vi "open_dev3.vi"(4 "ViStatus":T2, 7 "InterfaceInfo 2":T3) -> (0 "ViStatus 2":T2, 1 "drv_name":string, 2 "ModuleInfo":T1 {"DacScaleCoef" format="%#_2g"; "DacOffsetCoef" format="%#_2g"}, 3 "InterfaceInfo":T3)   [LabVIEW 2010]
uses:
  Rtusbapi.llb/3000pars.vi
  wrRtusbapi.dll
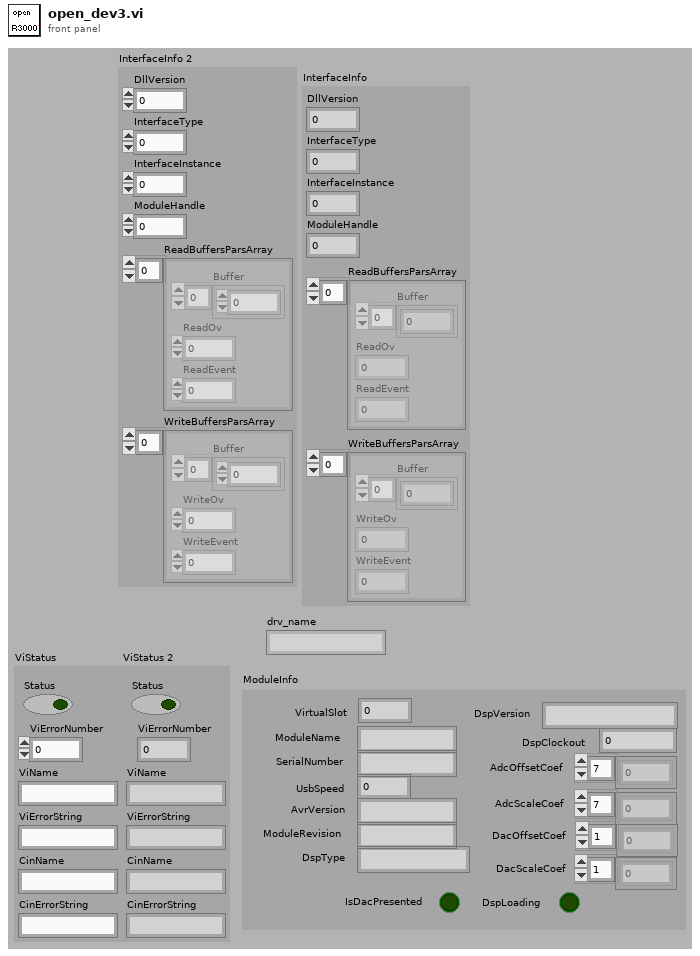
[diagram p1: front panel]
types:
  T1 = cluster{"VirtualSlot":u16, "ModuleName":string, "SerialNumber":string, "UsbSpeed":u8, "AvrVersion":string, "ModuleRevision":string, "DspType":string, "IsDacPresented":bool, "DspLoading":bool, "DspVersion":string, "DspClockout":u32, "AdcOffsetCoef":sgl[], "AdcScaleCoef":sgl[], "DacOffsetCoef":sgl[], "DacScaleCoef":sgl[]}
  T2 = cluster{"Status":bool, "ViErrorNumber":u32, "ViName":string, "ViErrorString":string, "CinName":string, "CinErrorString":string}
  T3 = cluster{"DllVersion":u32, "InterfaceType":u32, "InterfaceInstance":u32, "ModuleHandle":u32, "ReadBuffersParsArray":cluster{"Buffer":i16[], "ReadOv":u32, "ReadEvent":u32}[], "WriteBuffersParsArray":cluster{"Buffer":i16[], "WriteOv":u32, "WriteEvent":u32}[]}
  T4 = cluster{"CRC16":u16, "size":u16, "SerialNumber":string, "Name":string, "Revision":string, "DSPType":string, "IsDACPresent":u16, "DSPClockout":u32, "ADCOffset":sgl[], "ADCScale":sgl[], "DACOffset":sgl[], "DACScale":sgl[]}
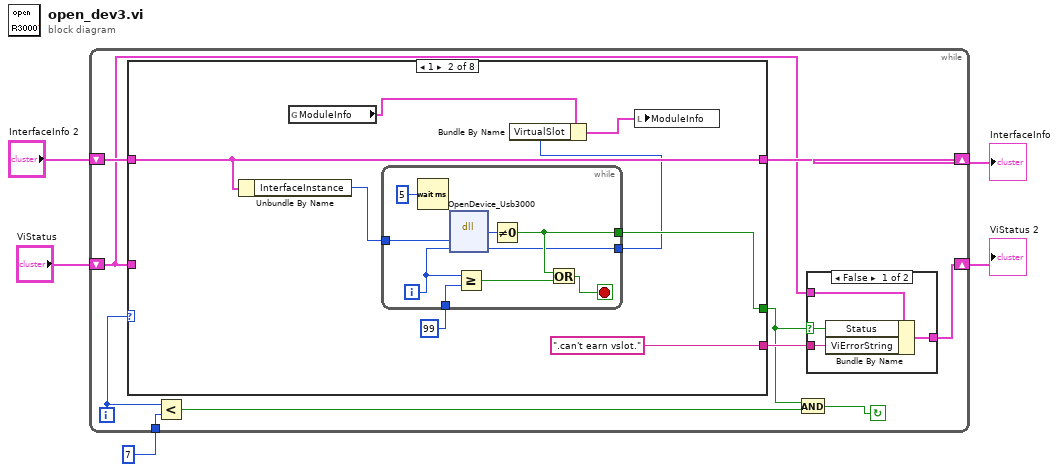
[diagram p0: block diagram]
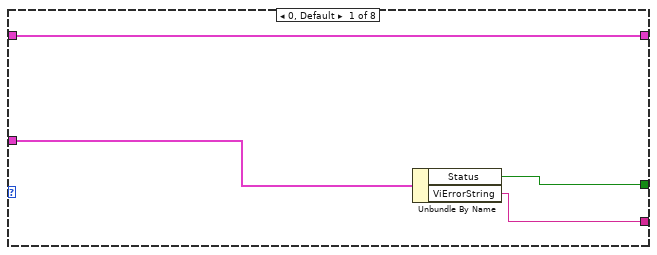
[diagram p3: hidden frame]
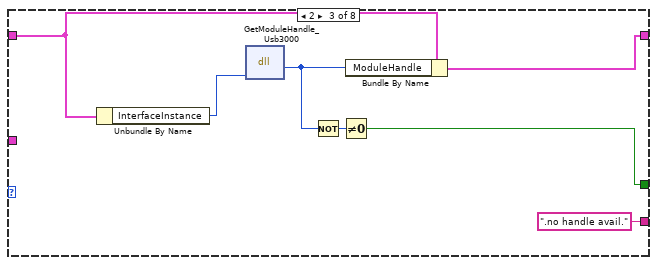
[diagram p4: hidden frame]
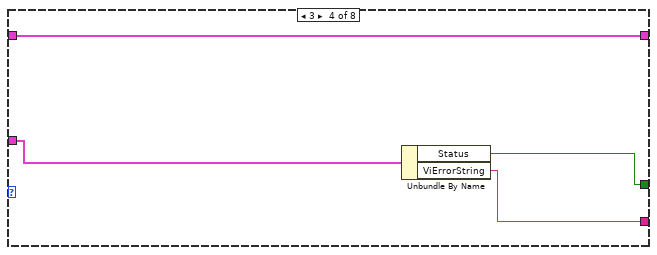
[diagram p5: hidden frame]
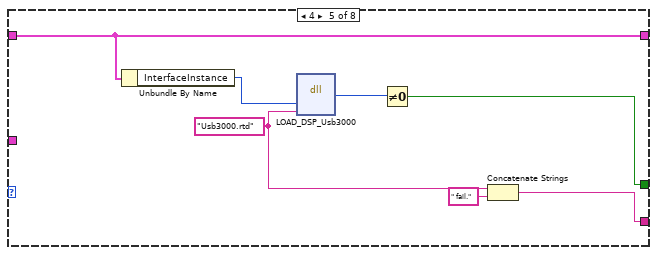
[diagram p6: hidden frame]
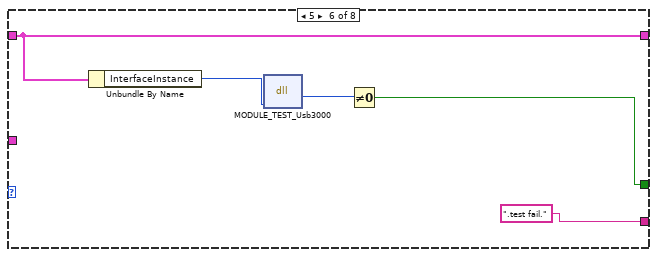
[diagram p7: hidden frame]
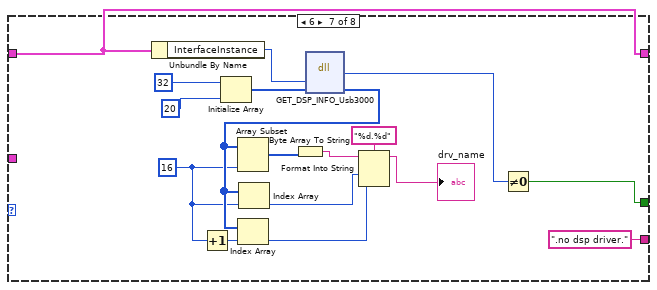
[diagram p8: hidden frame]
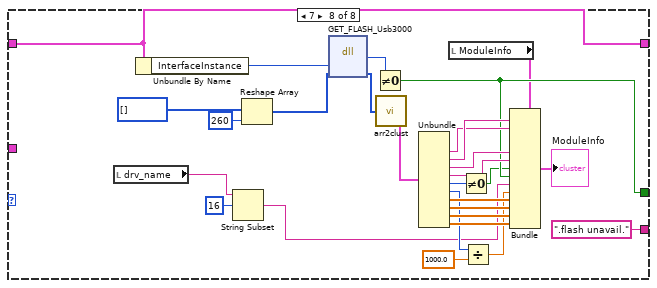
[diagram p9: hidden frame]
diagram:
  n1 = while {
    shift-right: [w14] -> w3
    shift-left: "InterfaceInfo 2" -> [w15]
    shift-right: [w12] -> w2
    shift-left: "ViStatus" -> [w13]
    tunnel: 7 ("y") -> [w6]
    i -> [w10]
    stop <- w7 continue-if-true
    n2 = case shown="1" w10 {
      tunnel: w15 -> [w24 w31 w47 w52 w59 w61 w78 w109]
      tunnel: [w24 w31 w46 w52 w59 w61 w78 w109] -> w14
      tunnel: w13 -> [w23 _ _ w50 _ _ _ _]
      tunnel: [w22 w30 w44 w51 w56 w62 w75 w95] -> w9
      tunnel: [w21 ".can't earn vslot." ("ViErrorString") ".no handle avail." ("ViErrorString") w49 w54 ".test fail." ("ViErrorString") ".no dsp driver." ("ViErrorString") ".flash unavail." ("ViErrorString")] -> w11
      frame 0, Default {
        n3 = Unbundle By Name(w23) -> ("Status"=w22:bool, "ViErrorString"=w21:string)
      }
      frame 1 {
        n4 = Unbundle By Name(w31) -> ("InterfaceInstance"=w32:u32)
        n5 = global read "3000pars.vi" "ModuleInfo"() -> (w26:T1)
        n6 = while {
          tunnel: w32 -> [w41]
          tunnel: [w37] -> w30
          tunnel: 99 -> [w38]
          tunnel: [w34] -> w27
          i -> [w39]
          stop <- w36 stop-if-true
          n7 = Wait (ms)(milliseconds to wait=u32 5) -> ()  [unwired: 1 out]
          n8 = dll-call lib="D:/Work/SibNIIE/SMGR/prj1_pdv_usb/pdv_usb/wrRtusbapi.dll" fn="OpenDevice_Usb3000"(w41, w39) -> (w40:i32, w34:u16)  [unwired: 4 in, 2 out]
          n9 = Greater Or Equal?(x=w39, y=w38) -> (x >= y?=w35:bool)
          n10 = Not Equal To 0?(x=w40) -> (x != 0?=w37:bool)
          n11 = Or(x=w37, y=w35) -> (x .or. y?=w36:bool)
        }
        n12 = Bundle By Name(cluster=w26, "VirtualSlot"=w27) -> (w25:T1)
        n13 = local write "ModuleInfo"(w25) -> ()
      }
      frame 2 {
        n14 = Unbundle By Name(w47) -> ("InterfaceInstance"=w48:u32)
        n15 = dll-call lib="D:/Work/SibNIIE/SMGR/prj1_pdv_usb/pdv_usb/wrRtusbapi.dll" fn="GetModuleHandle_Usb3000"(w48) -> (w42:u32)  [unwired: 4 in, 2 out]
        n16 = Not(x=w42) -> (.not. x?=w45:u32)
        n17 = Not Equal To 0?(x=w45) -> (x != 0?=w44:bool)
        n18 = Bundle By Name(cluster=w47, "ModuleHandle"=w42) -> (w46:T3)
      }
      frame 3 {
        n19 = Unbundle By Name(w50) -> ("Status"=w51:bool, "ViErrorString"=w49:string)
      }
      frame 4 {
        w55 = "Usb3000.rtd" ("input param")
        n20 = Unbundle By Name(w59) -> ("InterfaceInstance"=w58:u32)
        n21 = dll-call lib="D:/Work/SibNIIE/SMGR/prj1_pdv_usb/pdv_usb/wrRtusbapi.dll" fn="LOAD_DSP_Usb3000"(w58, w55) -> (w57:i32)  [unwired: 5 in, 2 out]
        n22 = Not Equal To 0?(x=w57) -> (x != 0?=w56:bool)
        n23 = Concatenate Strings(w55, " fail." ("string")) -> (w54:string)
      }
      frame 5 {
        n24 = Unbundle By Name(w61) -> ("InterfaceInstance"=w64:u32)
        n25 = dll-call lib="D:/Work/SibNIIE/SMGR/prj1_pdv_usb/pdv_usb/wrRtusbapi.dll" fn="MODULE_TEST_Usb3000"(w64) -> (w63:i32)  [unwired: 4 in, 2 out]
        n26 = Not Equal To 0?(x=w63) -> (x != 0?=w62:bool)
      }
      frame 6 {
        w65 = 16 ("length")
        n27 = Unbundle By Name(w78) -> ("InterfaceInstance"=w77:u32)
        n28 = Increment(x=w65) -> (x+1=w66:i32)
        n29 = Initialize Array(u8 32, 20) -> (w81:u8[])
        n30 = dll-call lib="D:/Work/SibNIIE/SMGR/prj1_pdv_usb/pdv_usb/wrRtusbapi.dll" fn="GET_DSP_INFO_Usb3000"(w77, w81) -> (w76:i32, w71:u8[])  [unwired: 4 in, 2 out]
        n31 = Array Subset(array=w71, length=w65) -> (w73:u8[])  [unwired: 1 in]
        n32 = Index Array(array=w71, index=w66) -> (element=w69:u8)
        n33 = Index Array(array=w71, index=w65) -> (element=w70:u8)
        n34 = Byte Array To String(unsigned byte array=w73) -> (string=w72:string)
        n35 = Format Into String(format string="%d.%d", initial string=w72, w70, w69) -> (resulting string=→"drv_name":string)  [unwired: 1 in, 1 out]
        n36 = Not Equal To 0?(x=w76) -> (x != 0?=w75:bool)
      }
      frame 7 {
        n37 = local read "drv_name"() -> (w84:string)
        n38 = Unbundle By Name(w109) -> ("InterfaceInstance"=w107:u32)
        n39 = String Subset(string=w84, offset (0)=16) -> (substring=w83:string)  [unwired: 1 in]
        n40 = Reshape Array(u8[] [] ("input param"), 260 ("dimension size")) -> (w105:u8[])
        n41 = dll-call lib="D:/Work/SibNIIE/SMGR/prj1_pdv_usb/pdv_usb/wrRtusbapi.dll" fn="GET_FLASH_Usb3000"(w107, w105) -> (w108:i32, w102:u8[])  [unwired: 4 in, 2 out]
        n42 = Not Equal To 0?(x=w108) -> (x != 0?=w95:bool)
        n43 = call "arr2clust.vi"("Array"=w102) -> ("Cluster"=w101:T4)
        n44 = Unbundle(w101) -> ("SerialNumber"=w98:string, "Name"=w99:string, "Revision"=w97:string, "DSPType"=w96:string, "IsDACPresent"=w90:u16, "DSPClockout"=w87:u32, "ADCOffset"=w94:sgl[], "ADCScale"=w93:sgl[], "DACOffset"=w92:sgl[], "DACScale"=w91:sgl[])  [unwired: 2 out]
        n45 = local read "ModuleInfo"() -> (w82:T1)
        n46 = Not Equal To 0?(x=w90) -> (x != 0?=w89:bool)
        n47 = Divide(x=w87, y=1000.0) -> (x/y=w86:dbl)
        n48 = Bundle(cluster=w82, "ModuleName"=w99, "SerialNumber"=w98, "ModuleRevision"=w97, "DspType"=w96, "IsDacPresented"=w89, "DspLoading"=w95, "DspVersion"=w83, "DspClockout"=w86, "AdcOffsetCoef"=w94, "AdcScaleCoef"=w93, "DacOffsetCoef"=w92, "DacScaleCoef"=w91) -> (→"ModuleInfo":T1)  [unwired: 3 in]
      }
    }
    n49 = Less?(x=w10, y=w6) -> (x < y?=w8:bool)
    n50 = And(x=w9, y=w8) -> (x .and. y?=w7:bool)
    n51 = case shown="False" w9 {
      selector: w9 -> [w16 _]
      tunnel: w13 -> [w19 w20]
      tunnel: [w18 w20] -> w12
      tunnel: w11 -> [w17 _]
      frame False {
        n52 = Bundle By Name(cluster=w19, "Status"=w16, "ViErrorString"=w17) -> (w18:T2)
      }
      frame True {
        # "ok"
      }
    }
  }
  "InterfaceInfo" <- w3
  "ViStatus 2" <- w2
